vi "RESTful API_old.vi"(4 "data":T3[](array[typedef]), 6 "Method":T2(ring), 7 "url":string, 8 "error in":errorcluster, 9 "JSON":string, 11 "Device In":T4={"Name"="", "BaseURL"="", "AppKey"="", "Headers"=["Content-Type:application/json"], "Timeout"=10000}) -> (0 "error out":errorcluster, 2 "Comm":T1, 3 "Device Out":T4={"Name"="", "BaseURL"="", "AppKey"="", "Headers"=["Content-Type:application/json"], "Timeout"=10000})   [LabVIEW 2020]
uses:
  <vilib>/httpClient/MultipartData.ctl
  <vilib>/httpClient/PUTBuffer.vi
  <vilib>/httpClient/POSTBuffer.vi
  <vilib>/httpClient/LabVIEWHTTPClient.lvlib
panel:
  out "HTTP Code":i32
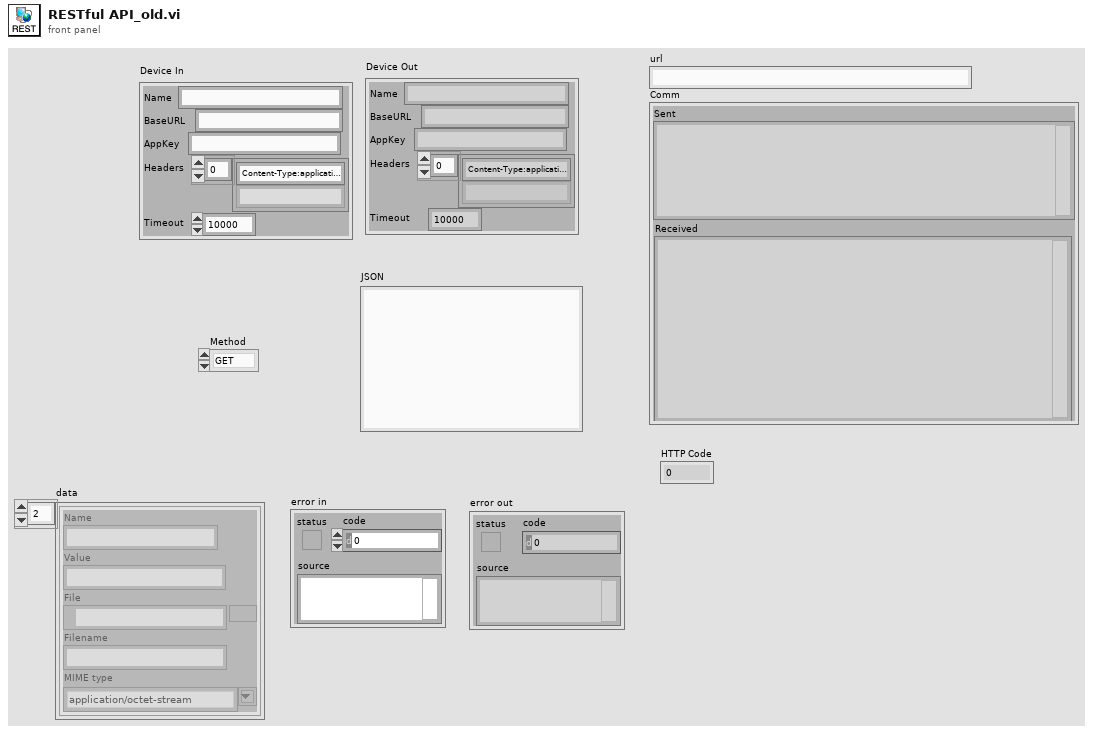
[diagram p1: front panel]
types:
  T1 = cluster{"url":string, "sent headers":string, "sent body":string, "headers":string, "body":string, "Sent":string, "Received":string}
  T2 = enum16{"GET", "PUT", "POST", "MultiPOST", "DELETE"}
  T3 = typedef "LabVIEWHTTPClient.lvlib/MultipartData.ctl" = cluster{"Name":string, "Value":string, "File":path, "Filename":string, "MIME type":string}
  T4 = cluster{"Name":string, "BaseURL":string, "AppKey":string, "Headers":string[], "Timeout":i32}
  T5 = typedef "LabVIEWHTTPClient.lvlib/ClientHandle.ctl" = refnum<k1>
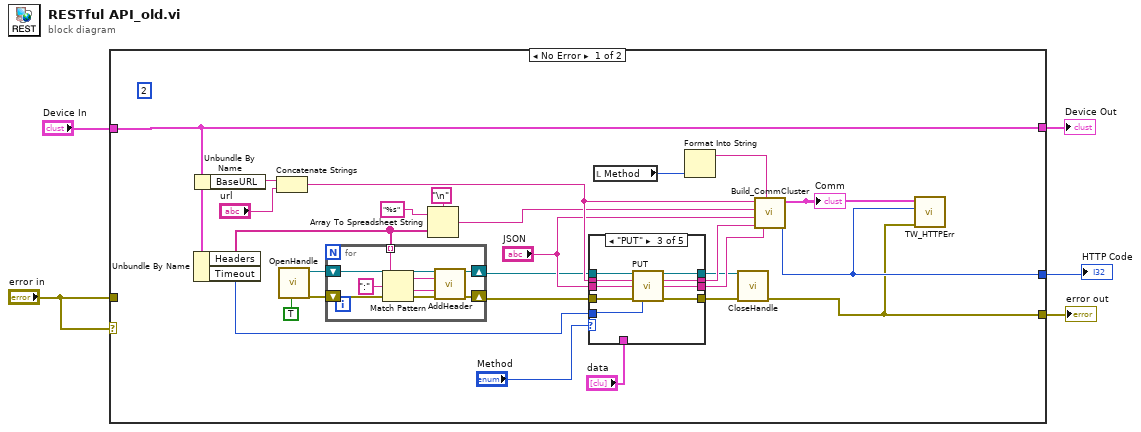
[diagram p0: block diagram]
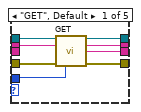
[diagram p2: hidden frame]
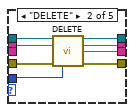
[diagram p3: hidden frame]
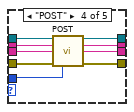
[diagram p4: hidden frame]
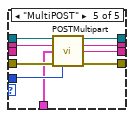
[diagram p5: hidden frame]
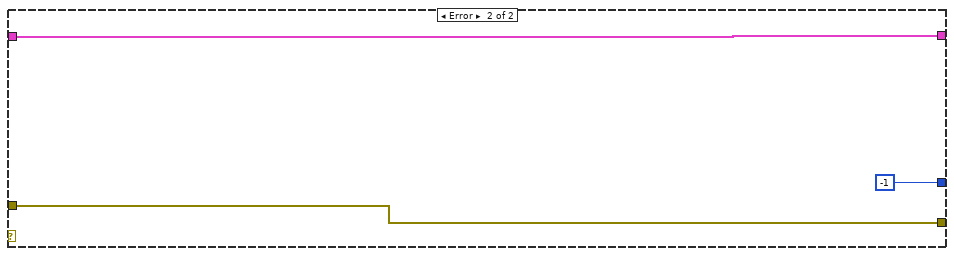
[diagram p6: hidden frame]
diagram:
  n1 = case shown="No Error" "error in" {
    tunnel: "error in" -> [_ w84]
    tunnel: "Device In" -> [w9 w85]
    tunnel: [w9 w85] -> w4
    tunnel: [w6 w84] -> w3
    tunnel: [w7 -1 ("error")] -> w1
    frame No Error {
      (unwired) 2
      n2 = Unbundle By Name(w9) -> ("Headers"=w18:string[], "Timeout"=w19:i32)
      n3 = Unbundle By Name(w9) -> ("BaseURL"=w27:string)
      n4 = Concatenate Strings(w27, "url") -> (w30:string)
      n5 = call <vilib>:"OpenHandle.vi"("verify server(true)"=TRUE) -> ("client handle out"=w21:T5, "error out"=w22:errorcluster)  [unwired: 13 in]
      n6 = for {
        shift-right: [w38] -> w14
        shift-left: w21 -> [w39]
        shift-right: [w36] -> w13
        shift-left: w22 -> [w37]
        tunnel: w18 -> [w32] mode=indexing
        n7 = Match Pattern(string=w32, regular expression=":") -> (before substring=w34:string, after substring=w33:string)  [unwired: 1 in, 2 out]
        n8 = call <vilib>:"AddHeader.vi"("client handle"=w39, "header"=w34, "value"=w33, "error in (no error)"=w37) -> ("client handle out"=w38:T5, "error out"=w36:errorcluster)  [unwired: 10 in]
      }
      n9 = Array To Spreadsheet String(delimiter (Tab)="\n", array=w18, 3:"%s" ("format string")) -> (spreadsheet string=w15:string)
      n10 = case shown="\"PUT\"" "Method" {
        tunnel: [w47 w55 w64 w73 w82] -> w31
        tunnel: [w46 w54 w63 w72 w81] -> w12
        tunnel: [w45 w53 w62 w71 w80] -> w10
        tunnel: w19 -> [w44 w52 w61 w70 w79]
        tunnel: w30 -> [w43 w51 w60 w69 w78]
        tunnel: w13 -> [w42 w50 w59 w68 w77]
        tunnel: w14 -> [w41 w49 w58 w67 w76]
        tunnel: "JSON" -> [_ _ w57 w66 _]
        tunnel: [w40 w48 w56 w65 w75] -> w11
        tunnel: "data" -> [_ _ _ _ w74]
        frame "GET", Default {
          n11 = call <vilib>:"GET.vi"("client handle"=w41, "url"=w43, "error in (no error)"=w42, "timeout (10000)"=w44) -> ("client handle out"=w40:T5, "headers"=w47:string, "body"=w46:string, "error out"=w45:errorcluster)  [unwired: 8 in]
        }
        frame "DELETE" {
          n12 = call <vilib>:"DELETE.vi"("client handle"=w49, "url"=w51, "error in (no error)"=w50, "timeout (10000)"=w52) -> ("client handle out"=w48:T5, "headers"=w55:string, "body"=w54:string, "error out"=w53:errorcluster)  [unwired: 8 in]
        }
        frame "PUT" {
          n13 = call-poly <vilib>:"PUT.vi"("client handle"=w58, "url"=w60, "buffer"=w57, "error in (no error)"=w59, "timeout (10000)"=w61) -> ("client handle out"=w56:T5, "headers"=w64:string, "body"=w63:string, "error out"=w62:errorcluster)  [unwired: 7 in]
        }
        frame "POST" {
          n14 = call-poly <vilib>:"POST.vi"("client handle"=w67, "url"=w69, "buffer"=w66, "error in (no error)"=w68, "timeout (10000)"=w70) -> ("client handle out"=w65:T5, "headers"=w73:string, "body"=w72:string, "error out"=w71:errorcluster)  [unwired: 7 in]
        }
        frame "MultiPOST" {
          n15 = call <vilib>:"POSTMultipart.vi"("client handle"=w76, "url"=w78, "data"=w74, "error in (no error)"=w77, "timeout (10000)"=w79) -> ("client handle out"=w75:T5, "headers"=w82:string, "body"=w81:string, "error out"=w80:errorcluster)  [unwired: 7 in]
        }
      }
      n16 = local read "Method"() -> (w25:T2)
      n17 = Format Into String(w25) -> (resulting string=w24:string)  [unwired: 3 in, 1 out]
      n18 = call <vilib>:"CloseHandle.vi"("client handle"=w11, "error in (no error)"=w10) -> ("error out"=w6:errorcluster)  [unwired: 13 in]
      n19 = call "Build_CommCluster.vi"("reply body"=w12, "Type"=w24, "reply headers"=w31, "sent body"="JSON", "sent headers"=w15, "url"=w30) -> ("Code"=w7:i32, "Comm"=w8:T1)  [unwired: 4 in]
      "Comm" <- w8
      n20 = call "TW_HTTPErr.vi"("error in (no error)"=w6, "HTTP Code"=w7, "Comm"=w8) -> ()  [unwired: 9 in]
    }
    frame Error {
    }
  }
  "error out" <- w3
  "Device Out" <- w4
  "HTTP Code" <- w1
